vi "init.vi"(8 "error in (no error)":errorcluster, 11 "hardware in":refnum<class "hardware.lvclass">) -> (0 "error out":errorcluster, 3 "hardware out":refnum<class "hardware.lvclass">)   [LabVIEW 2025, in "hardware.lvclass"]
uses:
  hardware.lvclass
  hardware.lvclass/hardware.ctl
  <vilib>/DAQmx/create/channels.llb/DAQmx Create Channel (AI-Temperature-Thermocouple).vi
  <vilib>/DAQmx/create/channels.llb/DAQmx Create Channel (DO-Digital Output).vi
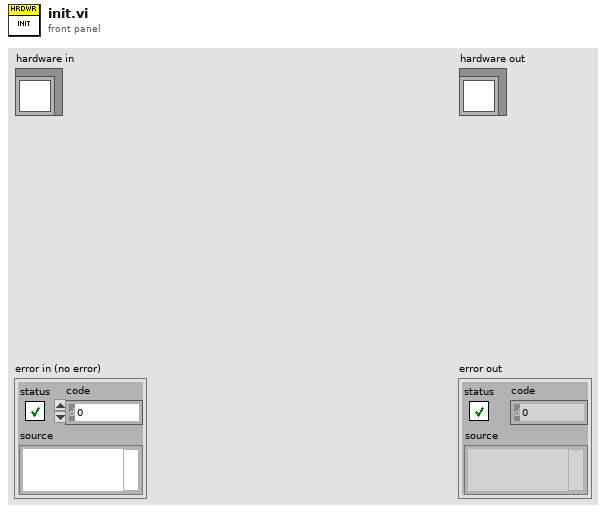
[diagram p1: front panel]
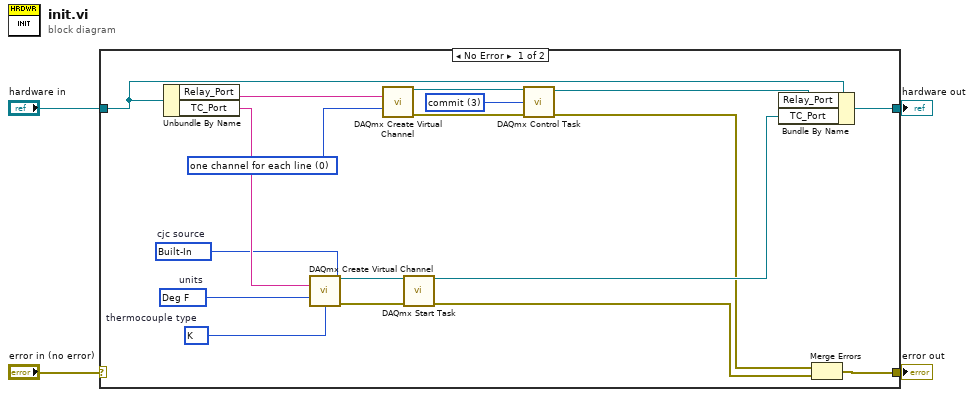
[diagram p0: block diagram]
diagram:
  n1 = case shown="No Error" "error in (no error)" {
    selector: "error in (no error)" -> [_ w24]
    tunnel: [w8 w24] -> w3
    tunnel: [w16 w23] -> w1
    tunnel: "hardware in" -> [w5 w23]
    frame No Error {
      w10 = 3 items=["verify"=2, "reserve"=4, "commit"=3, "unreserve"=5, "abort"=6] ("action")
      w13 = 0 items=["one channel for each line", "one channel for all lines"] ("line grouping")
      w19 = 10200 items=["Built-In"=10200, "Constant Value"=10116, "Channel"=10113]  # cjc source
      w20 = 10073 items=["J"=10072, "K"=10073, "N"=10077, "R"=10082, "S"=10085, "T"=10086, "B"=10047, "E"=10055, "A"=16208, "C"=16209]  # thermocouple type
      w21 = 10144 items=["Deg C"=10143, "Deg F"=10144, "Kelvins"=10325, "Deg R"=10145, "From Custom Scale"=10065]  # units
      n2 = Unbundle By Name(w5) -> ("Relay_Port"=w14:string, "TC_Port"=w22:string)
      n3 = call-poly <vilib>:"DAQmx Create Virtual Channel.vi"("physical channels"=w22, "cjc source"=w19, "units"=w21, "thermocouple type"=w20) -> ("task out"=w18:refnum<k21>, "error out"=w17:errorcluster)  [unwired: 10 in]
      n4 = call-poly <vilib>:"DAQmx Create Virtual Channel.vi"("lines"=w14, "line grouping"=w13) -> ("task out"=w12:refnum<k21>, "error out"=w11:errorcluster)  [unwired: 12 in]
      n5 = call <vilib>:"DAQmx Start Task.vi"("task/channels in"=w18, "error in"=w17) -> ("task out"=w15:refnum<k21>, "error out"=w6:errorcluster)  [unwired: 12 in]
      n6 = call <vilib>:"DAQmx Control Task.vi"("task/channels in"=w12, "action"=w10, "error in"=w11) -> ("task out"=w9:refnum<k21>, "error out"=w7:errorcluster)  [unwired: 11 in]
      n7 = Bundle By Name(cluster=w5, "Relay_Port"=w9, "TC_Port"=w15) -> (w16:refnum<class "hardware.lvclass">)
      n8 = Merge Errors(w7, w6) -> (w8:errorcluster)
    }
    frame Error {
    }
  }
  "error out" <- w3
  "hardware out" <- w1
